vi "Instructor Read Client.vi"() -> ()   [LabVIEW 2017]
uses:
  <vilib>/OPCUA/controls/NodeIds.ctl
  <vilib>/OPCUA/controls/NodeId.ctl
  <vilib>/OPCUA/NI OPC UA Client.lvlib
panel:
  in  "stop":bool
  out "error out":errorcluster
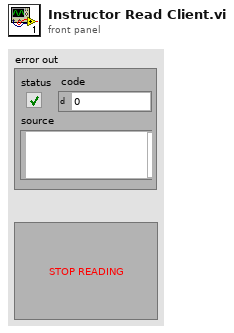
[diagram p1: front panel]
types:
  T1 = cluster{"message mode":enum16{"None", "Sign", "Sign and Encrypt"}, "security":enum16{"Basic256", "Basic128Rsa15"}}
  T2 = typedef "NodeIds.ctl" = T3[]
  T3 = typedef "NodeId.ctl" = string
  T4 = typedef "OPC UA Client Refnum.ctl" = refnum<k21>
  T5 = typedef "Subscription ID.ctl" = u32
  T6 = typedef "Subscription Data Change.ctl" = cluster{"node ID":T3, " value":variant, "timestamp":timestamp, "data type":T7, "status code":T8}
  T7 = typedef "Data Type.ctl" = u16
  T8 = typedef "OPC UA StatusCode.ctl" = u32
  T9 = cluster{"[0]":sgl, "[1]":sgl, "[2]":sgl, "[3]":sgl, "[4]":sgl, "[5]":sgl, "[6]":sgl, "[7]":sgl, "[8]":sgl, "[9]":sgl, "[10]":sgl, "[11]":sgl, "[12]":sgl, "[13]":sgl, "[14]":sgl, "[15]":sgl, "[16]":sgl, "[17]":sgl, "[18]":sgl, "[19]":sgl, "[20]":sgl, "[21]":sgl, "[22]":sgl, "[23]":sgl, "[24]":sgl, "[25]":sgl, "[26]":sgl, "[27]":sgl, "[28]":sgl, "[29]":sgl, "[30]":sgl, "[31]":sgl, "[32]":sgl, "[33]":sgl, "[34]":sgl, "[35]":sgl, "[36]":sgl, "[37]":sgl, "[38]":sgl, "[39]":sgl, "[40]":sgl, "[41]":sgl, "[42]":sgl, "[43]":sgl, "[44]":sgl, "[45]":sgl, "[46]":sgl, "[47]":sgl, "[48]":sgl, "[49]":sgl, "[50]":sgl, "[51]":sgl, "[52]":sgl, "[53]":sgl, "[54]":sgl, "[55]":sgl, "[56]":sgl, "[57]":sgl, "[58]":sgl, "[59]":sgl, "[60]":sgl, "[61]":sgl, "[62]":sgl}
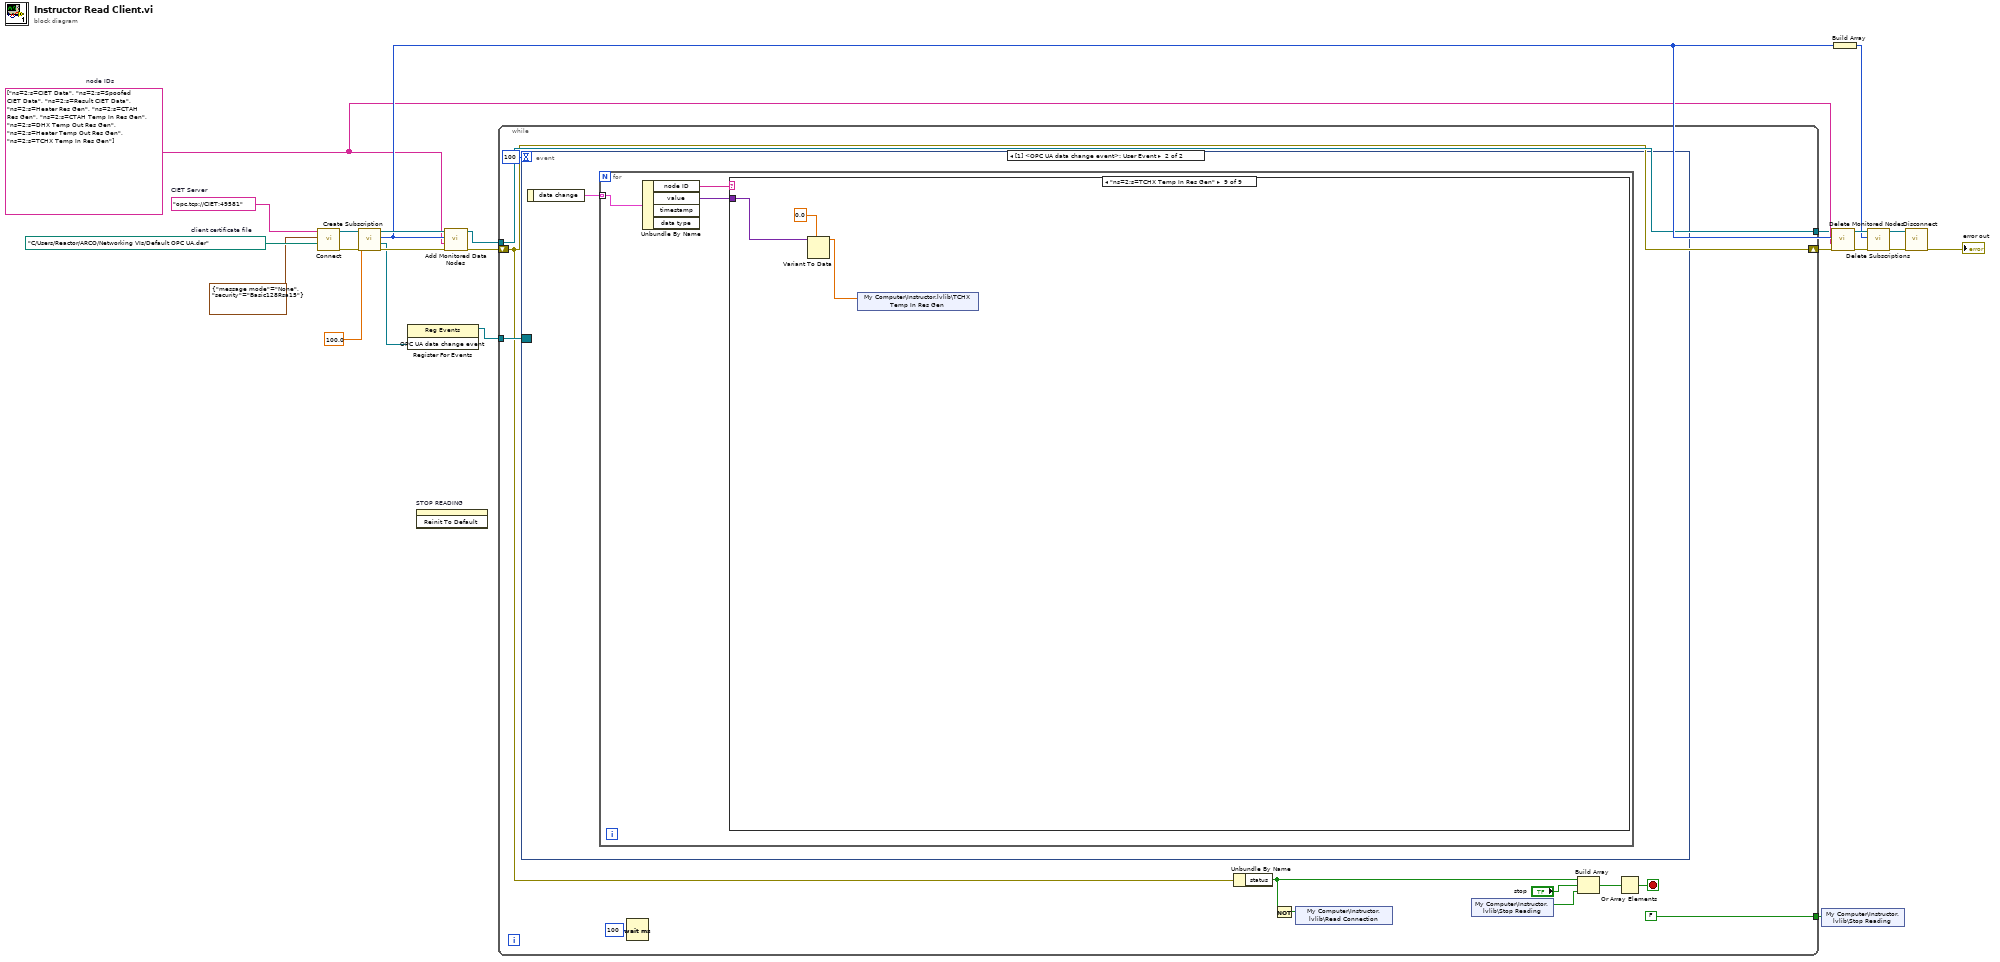
[diagram p0: block diagram]
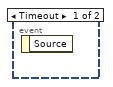
[diagram p2: hidden frame]
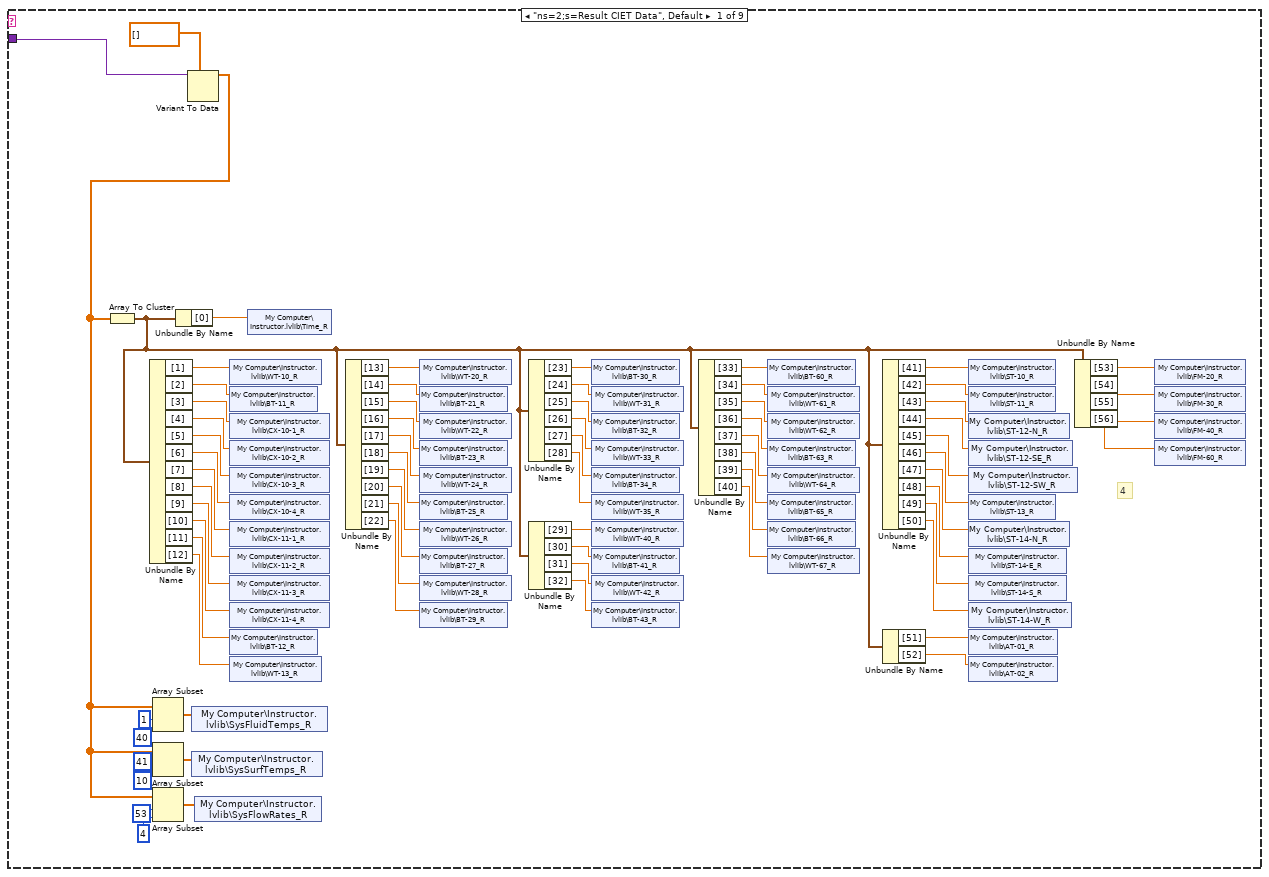
[diagram p3: hidden frame]
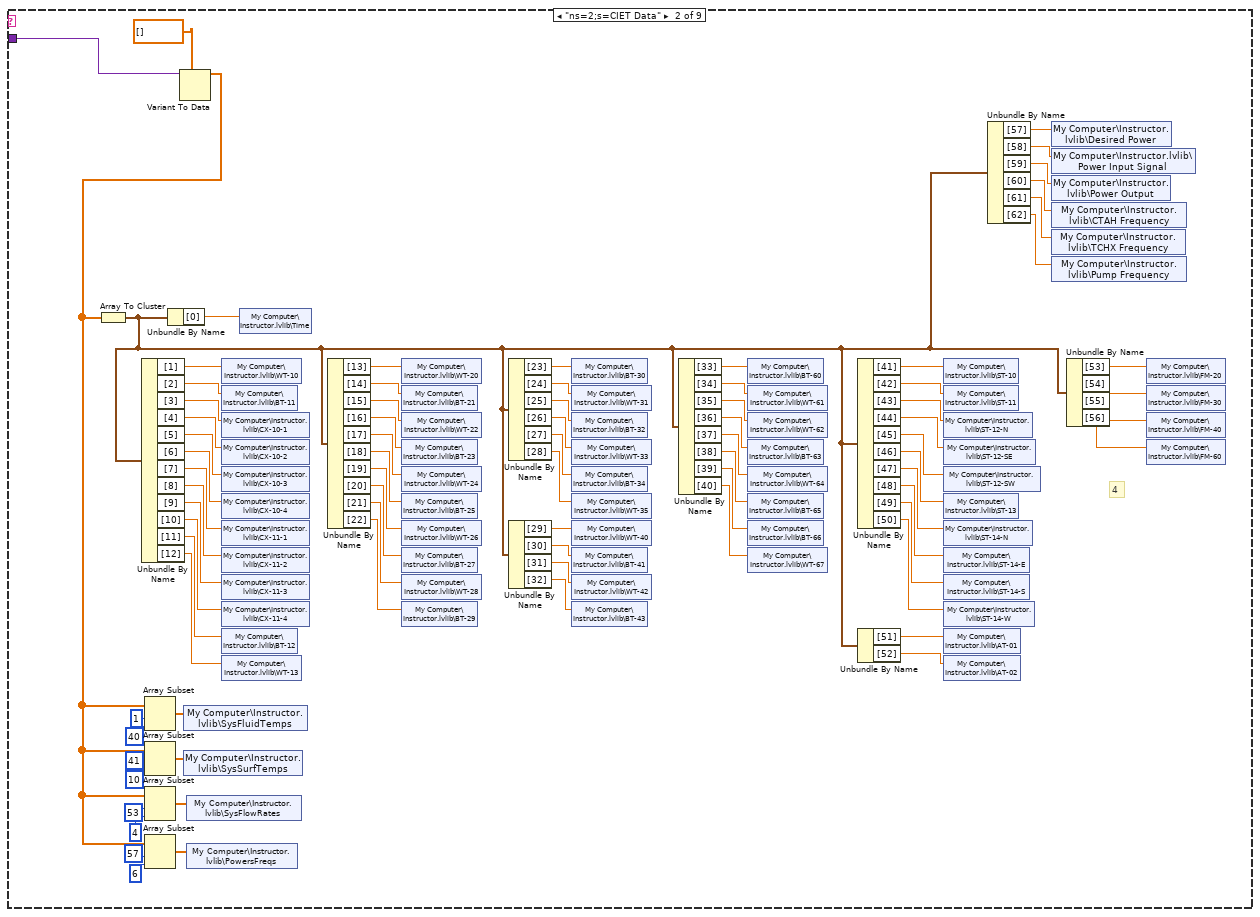
[diagram p4: hidden frame]
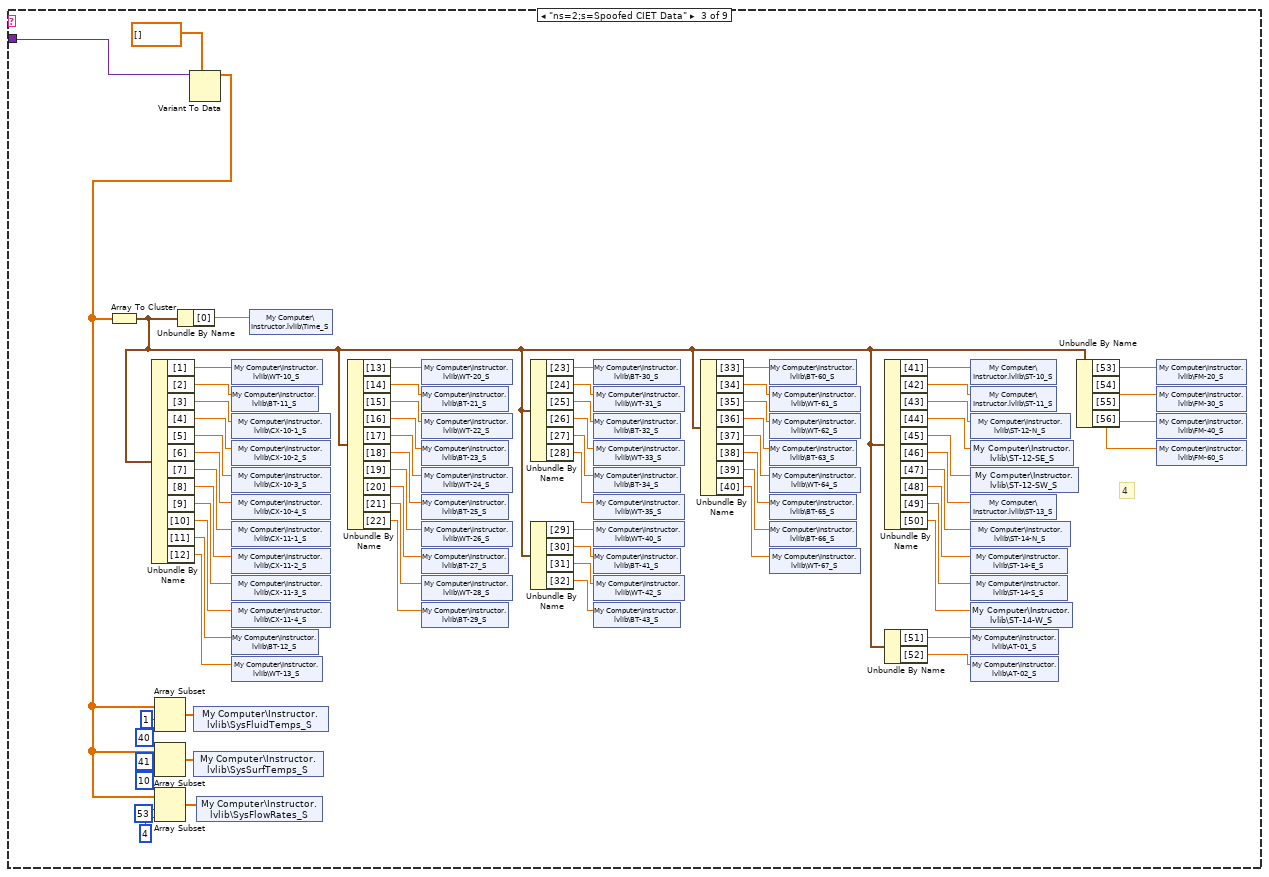
[diagram p5: hidden frame]
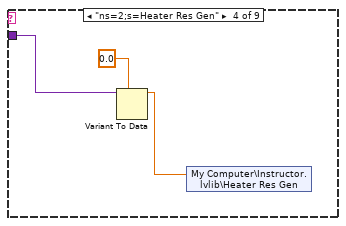
[diagram p6: hidden frame]
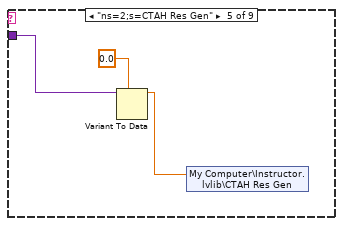
[diagram p7: hidden frame]
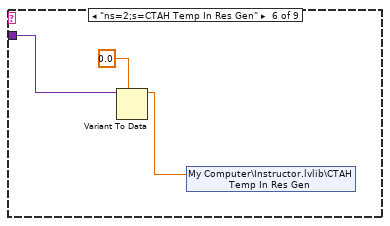
[diagram p8: hidden frame]
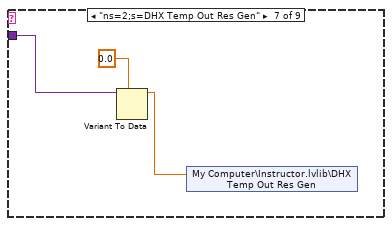
[diagram p9: hidden frame]
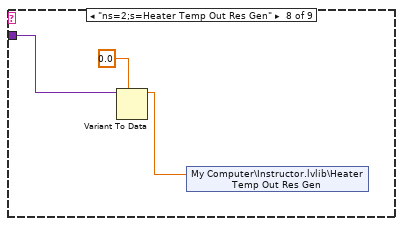
[diagram p10: hidden frame]
diagram:
  w7 = T2 ["ns=2;s=CIET Data", "ns=2;s=Spoofed CIET Data", "ns=2;s=Result CIET Data", "ns=2;s=Heater Res Gen", "ns=2;s=CTAH Res Gen", "ns=2;s=CTAH Temp In Res Gen", "ns=2;s=DHX Temp Out Res Gen", "ns=2;s=Heater Temp Out Res Gen", "ns=2;s=TCHX Temp In Res Gen"]  # node IDs
  w21 = path "C:/Users/Reactor/ARCO/Networking VIs/Default OPC UA.der"  # client certificate file
  w22 = "opc.tcp://CIET:49581"  # CIET Server
  n1 = call <vilib>:"Connect.vi"("client certificate file"=w21, "security policy"=T1 {"message mode"=enum."None", "security"=enum."Basic128Rsa15"}, "server endpoint URL"=w22) -> ("error out"=w3:errorcluster, "OPC UA client refnum out"=w19:T4)  [unwired: 6 in, 1 out]
  n2 = call <vilib>:"Create Subscription.vi"("error in (no error)"=w3, "publishing interval (1000 ms)"=100.0, "OPC UA client refnum in"=w19) -> ("error out"=w17:errorcluster, "OPC UA data change event"=w16:refnum<user-event>, "subscription ID out"=w11:T5, "OPC UA client refnum out"=w18:T4)  [unwired: 4 in, 1 out]
  n3 = register-events(w16) -> (reference out=w9:refnum<event-registration>)  [unwired: 2 in, 1 out]
  n4 = invoke on="STOP READING" class="Bool (strict)" method="Reinit To Default"() -> ()  [unwired: 3 in, 3 out]
  n5 = call <vilib>:"Add Monitored Data Nodes.vi"("error in (no error)"=w17, "node IDs"=w7, "subscription ID in"=w11, "OPC UA client refnum in"=w18) -> ("error out"=w2:errorcluster, "OPC UA client refnum out"=w8:T4)  [unwired: 4 in, 2 out]
  n6 = while {
    tunnel: w9 -> [w35]
    tunnel: w8 -> [w33]
    tunnel: [w33] -> w6
    tunnel: [FALSE] -> w4
    shift-right: [w24] -> w1
    shift-left: w2 -> [w24]
    stop <- w25 stop-if-true
    n7 = event shown="[1] <OPC UA data change event>: User Event" {
      selector: w35 -> [_ _]
      dyn-events: _ -> [_ _]
      timeout: 100 -> [_ _]
      event Timeout {
        n8 = event-data() -> ()  [unwired: 1 in, 1 out]
      }
      event User Event {
        n9 = event-data() -> ("data change"=w36:T6[])  [unwired: 1 in]
        n10 = for {
          tunnel: w36 -> [w38] mode=indexing
          n11 = Unbundle By Name(w38) -> ("node ID"=w37:T3, "value"=w39:variant)  [unwired: 2 out]
          n12 = case shown="\"ns=2;s=TCHX Temp In Res Gen\"" w37 {
            tunnel: w39 -> [w43 w129 w191 w259 w262 w265 w268 w271 w274]
            frame "ns=2;s=Result CIET Data", Default {
              # "4"
              n13 = Variant To Data(type=sgl[] [], Variant=w43) -> (data=w41:sgl[])  [unwired: 1 in, 1 out]
              n14 = Array To Cluster(array=w41) -> (cluster=w40:T9)
              n15 = Unbundle By Name(w40) -> ("[1]"=w50:sgl, "[2]"=w52:sgl, "[3]"=w53:sgl, "[4]"=w54:sgl, "[5]"=w55:sgl, "[6]"=w56:sgl, "[7]"=w57:sgl, "[8]"=w58:sgl, "[9]"=w59:sgl, "[10]"=w60:sgl, "[11]"=w61:sgl, "[12]"=w62:sgl)
              n16 = Array Subset(array=w41, index=1, length=40) -> (w107:sgl[])
              n17 = Array Subset(array=w41, index=41, length=10) -> (w108:sgl[])
              n18 = Array Subset(array=w41, index=53, length=4) -> (w109:sgl[])
              n19 = Unbundle By Name(w40) -> ("[0]"=w51:sgl)
              n20 = shared-variable "My Computer\\Instructor.lvlib\\SysFluidTemps_R"(w107) -> ()  [unwired: 1 in, 1 out]
              n21 = shared-variable "My Computer\\Instructor.lvlib\\SysSurfTemps_R"(w108) -> ()  [unwired: 1 in, 1 out]
              n22 = shared-variable "My Computer\\Instructor.lvlib\\SysFlowRates_R"(w109) -> ()  [unwired: 1 in, 1 out]
              n23 = shared-variable "My Computer\\Instructor.lvlib\\WT-10_R"(w50) -> ()  [unwired: 1 in, 1 out]
              n24 = shared-variable "My Computer\\Instructor.lvlib\\BT-11_R"(w52) -> ()  [unwired: 1 in, 1 out]
              n25 = shared-variable "My Computer\\Instructor.lvlib\\CX-10-1_R"(w53) -> ()  [unwired: 1 in, 1 out]
              n26 = shared-variable "My Computer\\Instructor.lvlib\\CX-10-2_R"(w54) -> ()  [unwired: 1 in, 1 out]
              n27 = shared-variable "My Computer\\Instructor.lvlib\\CX-10-3_R"(w55) -> ()  [unwired: 1 in, 1 out]
              n28 = shared-variable "My Computer\\Instructor.lvlib\\CX-10-4_R"(w56) -> ()  [unwired: 1 in, 1 out]
              n29 = shared-variable "My Computer\\Instructor.lvlib\\CX-11-1_R"(w57) -> ()  [unwired: 1 in, 1 out]
              n30 = shared-variable "My Computer\\Instructor.lvlib\\CX-11-2_R"(w58) -> ()  [unwired: 1 in, 1 out]
              n31 = shared-variable "My Computer\\Instructor.lvlib\\CX-11-3_R"(w59) -> ()  [unwired: 1 in, 1 out]
              n32 = shared-variable "My Computer\\Instructor.lvlib\\CX-11-4_R"(w60) -> ()  [unwired: 1 in, 1 out]
              n33 = shared-variable "My Computer\\Instructor.lvlib\\BT-12_R"(w61) -> ()  [unwired: 1 in, 1 out]
              n34 = shared-variable "My Computer\\Instructor.lvlib\\WT-13_R"(w62) -> ()  [unwired: 1 in, 1 out]
              n35 = shared-variable "My Computer\\Instructor.lvlib\\Time_R"(w51) -> ()  [unwired: 1 in, 1 out]
              n36 = Unbundle By Name(w40) -> ("[13]"=w63:sgl, "[14]"=w64:sgl, "[15]"=w65:sgl, "[16]"=w66:sgl, "[17]"=w67:sgl, "[18]"=w68:sgl, "[19]"=w69:sgl, "[20]"=w70:sgl, "[21]"=w71:sgl, "[22]"=w72:sgl)
              n37 = shared-variable "My Computer\\Instructor.lvlib\\WT-20_R"(w63) -> ()  [unwired: 1 in, 1 out]
              n38 = shared-variable "My Computer\\Instructor.lvlib\\BT-21_R"(w64) -> ()  [unwired: 1 in, 1 out]
              n39 = shared-variable "My Computer\\Instructor.lvlib\\WT-22_R"(w65) -> ()  [unwired: 1 in, 1 out]
              n40 = shared-variable "My Computer\\Instructor.lvlib\\BT-23_R"(w66) -> ()  [unwired: 1 in, 1 out]
              n41 = shared-variable "My Computer\\Instructor.lvlib\\WT-24_R"(w67) -> ()  [unwired: 1 in, 1 out]
              n42 = shared-variable "My Computer\\Instructor.lvlib\\BT-25_R"(w68) -> ()  [unwired: 1 in, 1 out]
              n43 = shared-variable "My Computer\\Instructor.lvlib\\WT-26_R"(w69) -> ()  [unwired: 1 in, 1 out]
              n44 = shared-variable "My Computer\\Instructor.lvlib\\BT-27_R"(w70) -> ()  [unwired: 1 in, 1 out]
              n45 = shared-variable "My Computer\\Instructor.lvlib\\WT-28_R"(w71) -> ()  [unwired: 1 in, 1 out]
              n46 = shared-variable "My Computer\\Instructor.lvlib\\BT-29_R"(w72) -> ()  [unwired: 1 in, 1 out]
              n47 = Unbundle By Name(w40) -> ("[23]"=w73:sgl, "[24]"=w74:sgl, "[25]"=w75:sgl, "[26]"=w76:sgl, "[27]"=w77:sgl, "[28]"=w78:sgl)
              n48 = Unbundle By Name(w40) -> ("[29]"=w79:sgl, "[30]"=w80:sgl, "[31]"=w81:sgl, "[32]"=w82:sgl)
              n49 = shared-variable "My Computer\\Instructor.lvlib\\BT-30_R"(w73) -> ()  [unwired: 1 in, 1 out]
              n50 = shared-variable "My Computer\\Instructor.lvlib\\WT-31_R"(w74) -> ()  [unwired: 1 in, 1 out]
              n51 = shared-variable "My Computer\\Instructor.lvlib\\BT-32_R"(w75) -> ()  [unwired: 1 in, 1 out]
              n52 = shared-variable "My Computer\\Instructor.lvlib\\WT-33_R"(w76) -> ()  [unwired: 1 in, 1 out]
              n53 = shared-variable "My Computer\\Instructor.lvlib\\BT-34_R"(w77) -> ()  [unwired: 1 in, 1 out]
              n54 = shared-variable "My Computer\\Instructor.lvlib\\WT-35_R"(w78) -> ()  [unwired: 1 in, 1 out]
              n55 = shared-variable "My Computer\\Instructor.lvlib\\WT-40_R"(w79) -> ()  [unwired: 1 in, 1 out]
              n56 = shared-variable "My Computer\\Instructor.lvlib\\BT-41_R"(w80) -> ()  [unwired: 1 in, 1 out]
              n57 = shared-variable "My Computer\\Instructor.lvlib\\WT-42_R"(w81) -> ()  [unwired: 1 in, 1 out]
              n58 = shared-variable "My Computer\\Instructor.lvlib\\BT-43_R"(w82) -> ()  [unwired: 1 in, 1 out]
              n59 = Unbundle By Name(w40) -> ("[33]"=w83:sgl, "[34]"=w84:sgl, "[35]"=w85:sgl, "[36]"=w86:sgl, "[37]"=w87:sgl, "[38]"=w88:sgl, "[39]"=w89:sgl, "[40]"=w90:sgl)
              n60 = shared-variable "My Computer\\Instructor.lvlib\\BT-60_R"(w83) -> ()  [unwired: 1 in, 1 out]
              n61 = shared-variable "My Computer\\Instructor.lvlib\\WT-61_R"(w84) -> ()  [unwired: 1 in, 1 out]
              n62 = shared-variable "My Computer\\Instructor.lvlib\\WT-62_R"(w85) -> ()  [unwired: 1 in, 1 out]
              n63 = shared-variable "My Computer\\Instructor.lvlib\\BT-63_R"(w86) -> ()  [unwired: 1 in, 1 out]
              n64 = shared-variable "My Computer\\Instructor.lvlib\\WT-64_R"(w87) -> ()  [unwired: 1 in, 1 out]
              n65 = shared-variable "My Computer\\Instructor.lvlib\\BT-65_R"(w88) -> ()  [unwired: 1 in, 1 out]
              n66 = shared-variable "My Computer\\Instructor.lvlib\\BT-66_R"(w89) -> ()  [unwired: 1 in, 1 out]
              n67 = shared-variable "My Computer\\Instructor.lvlib\\WT-67_R"(w90) -> ()  [unwired: 1 in, 1 out]
              n68 = Unbundle By Name(w40) -> ("[41]"=w91:sgl, "[42]"=w92:sgl, "[43]"=w93:sgl, "[44]"=w94:sgl, "[45]"=w95:sgl, "[46]"=w96:sgl, "[47]"=w97:sgl, "[48]"=w98:sgl, "[49]"=w99:sgl, "[50]"=w100:sgl)
              n69 = Unbundle By Name(w40) -> ("[51]"=w101:sgl, "[52]"=w102:sgl)
              n70 = shared-variable "My Computer\\Instructor.lvlib\\ST-10_R"(w91) -> ()  [unwired: 1 in, 1 out]
              n71 = shared-variable "My Computer\\Instructor.lvlib\\ST-11_R"(w92) -> ()  [unwired: 1 in, 1 out]
              n72 = shared-variable "My Computer\\Instructor.lvlib\\ST-12-N_R"(w93) -> ()  [unwired: 1 in, 1 out]
              n73 = shared-variable "My Computer\\Instructor.lvlib\\ST-12-SE_R"(w94) -> ()  [unwired: 1 in, 1 out]
              n74 = shared-variable "My Computer\\Instructor.lvlib\\ST-12-SW_R"(w95) -> ()  [unwired: 1 in, 1 out]
              n75 = shared-variable "My Computer\\Instructor.lvlib\\ST-13_R"(w96) -> ()  [unwired: 1 in, 1 out]
              n76 = shared-variable "My Computer\\Instructor.lvlib\\ST-14-N_R"(w97) -> ()  [unwired: 1 in, 1 out]
              n77 = shared-variable "My Computer\\Instructor.lvlib\\ST-14-E_R"(w98) -> ()  [unwired: 1 in, 1 out]
              n78 = shared-variable "My Computer\\Instructor.lvlib\\ST-14-S_R"(w99) -> ()  [unwired: 1 in, 1 out]
              n79 = shared-variable "My Computer\\Instructor.lvlib\\ST-14-W_R"(w100) -> ()  [unwired: 1 in, 1 out]
              n80 = shared-variable "My Computer\\Instructor.lvlib\\AT-01_R"(w101) -> ()  [unwired: 1 in, 1 out]
              n81 = shared-variable "My Computer\\Instructor.lvlib\\AT-02_R"(w102) -> ()  [unwired: 1 in, 1 out]
              n82 = Unbundle By Name(w40) -> ("[53]"=w103:sgl, "[54]"=w104:sgl, "[55]"=w105:sgl, "[56]"=w106:sgl)
              n83 = shared-variable "My Computer\\Instructor.lvlib\\FM-20_R"(w103) -> ()  [unwired: 1 in, 1 out]
              n84 = shared-variable "My Computer\\Instructor.lvlib\\FM-30_R"(w104) -> ()  [unwired: 1 in, 1 out]
              n85 = shared-variable "My Computer\\Instructor.lvlib\\FM-40_R"(w105) -> ()  [unwired: 1 in, 1 out]
              n86 = shared-variable "My Computer\\Instructor.lvlib\\FM-60_R"(w106) -> ()  [unwired: 1 in, 1 out]
            }
            frame "ns=2;s=CIET Data" {
              # "4"
              n87 = Variant To Data(type=sgl[] [], Variant=w129) -> (data=w111:sgl[])  [unwired: 1 in, 1 out]
              n88 = Array To Cluster(array=w111) -> (cluster=w110:T9)
              n89 = Unbundle By Name(w110) -> ("[1]"=w128:sgl, "[2]"=w131:sgl, "[3]"=w132:sgl, "[4]"=w133:sgl, "[5]"=w134:sgl, "[6]"=w135:sgl, "[7]"=w136:sgl, "[8]"=w137:sgl, "[9]"=w138:sgl, "[10]"=w139:sgl, "[11]"=w140:sgl, "[12]"=w141:sgl)
              n90 = Array Subset(array=w111, index=1, length=40) -> (w186:sgl[])
              n91 = Array Subset(array=w111, index=41, length=10) -> (w187:sgl[])
              n92 = Array Subset(array=w111, index=53, length=4) -> (w188:sgl[])
              n93 = Array Subset(array=w111, index=57, length=6) -> (w118:sgl[])
              n94 = Unbundle By Name(w110) -> ("[0]"=w130:sgl)
              n95 = shared-variable "My Computer\\Instructor.lvlib\\SysFluidTemps"(w186) -> ()  [unwired: 1 in, 1 out]
              n96 = shared-variable "My Computer\\Instructor.lvlib\\SysSurfTemps"(w187) -> ()  [unwired: 1 in, 1 out]
              n97 = shared-variable "My Computer\\Instructor.lvlib\\SysFlowRates"(w188) -> ()  [unwired: 1 in, 1 out]
              n98 = shared-variable "My Computer\\Instructor.lvlib\\PowersFreqs"(w118) -> ()  [unwired: 1 in, 1 out]
              n99 = shared-variable "My Computer\\Instructor.lvlib\\WT-10"(w128) -> ()  [unwired: 1 in, 1 out]
              n100 = shared-variable "My Computer\\Instructor.lvlib\\BT-11"(w131) -> ()  [unwired: 1 in, 1 out]
              n101 = shared-variable "My Computer\\Instructor.lvlib\\CX-10-1"(w132) -> ()  [unwired: 1 in, 1 out]
              n102 = shared-variable "My Computer\\Instructor.lvlib\\CX-10-2"(w133) -> ()  [unwired: 1 in, 1 out]
              n103 = shared-variable "My Computer\\Instructor.lvlib\\CX-10-3"(w134) -> ()  [unwired: 1 in, 1 out]
              n104 = shared-variable "My Computer\\Instructor.lvlib\\CX-10-4"(w135) -> ()  [unwired: 1 in, 1 out]
              n105 = shared-variable "My Computer\\Instructor.lvlib\\CX-11-1"(w136) -> ()  [unwired: 1 in, 1 out]
              n106 = shared-variable "My Computer\\Instructor.lvlib\\CX-11-2"(w137) -> ()  [unwired: 1 in, 1 out]
              n107 = shared-variable "My Computer\\Instructor.lvlib\\CX-11-3"(w138) -> ()  [unwired: 1 in, 1 out]
              n108 = shared-variable "My Computer\\Instructor.lvlib\\CX-11-4"(w139) -> ()  [unwired: 1 in, 1 out]
              n109 = shared-variable "My Computer\\Instructor.lvlib\\BT-12"(w140) -> ()  [unwired: 1 in, 1 out]
              n110 = shared-variable "My Computer\\Instructor.lvlib\\WT-13"(w141) -> ()  [unwired: 1 in, 1 out]
              n111 = shared-variable "My Computer\\Instructor.lvlib\\Time"(w130) -> ()  [unwired: 1 in, 1 out]
              n112 = Unbundle By Name(w110) -> ("[13]"=w142:sgl, "[14]"=w143:sgl, "[15]"=w144:sgl, "[16]"=w145:sgl, "[17]"=w146:sgl, "[18]"=w147:sgl, "[19]"=w148:sgl, "[20]"=w149:sgl, "[21]"=w150:sgl, "[22]"=w151:sgl)
              n113 = shared-variable "My Computer\\Instructor.lvlib\\WT-20"(w142) -> ()  [unwired: 1 in, 1 out]
              n114 = shared-variable "My Computer\\Instructor.lvlib\\BT-21"(w143) -> ()  [unwired: 1 in, 1 out]
              n115 = shared-variable "My Computer\\Instructor.lvlib\\WT-22"(w144) -> ()  [unwired: 1 in, 1 out]
              n116 = shared-variable "My Computer\\Instructor.lvlib\\BT-23"(w145) -> ()  [unwired: 1 in, 1 out]
              n117 = shared-variable "My Computer\\Instructor.lvlib\\WT-24"(w146) -> ()  [unwired: 1 in, 1 out]
              n118 = shared-variable "My Computer\\Instructor.lvlib\\BT-25"(w147) -> ()  [unwired: 1 in, 1 out]
              n119 = shared-variable "My Computer\\Instructor.lvlib\\WT-26"(w148) -> ()  [unwired: 1 in, 1 out]
              n120 = shared-variable "My Computer\\Instructor.lvlib\\BT-27"(w149) -> ()  [unwired: 1 in, 1 out]
              n121 = shared-variable "My Computer\\Instructor.lvlib\\WT-28"(w150) -> ()  [unwired: 1 in, 1 out]
              n122 = shared-variable "My Computer\\Instructor.lvlib\\BT-29"(w151) -> ()  [unwired: 1 in, 1 out]
              n123 = Unbundle By Name(w110) -> ("[23]"=w152:sgl, "[24]"=w153:sgl, "[25]"=w154:sgl, "[26]"=w155:sgl, "[27]"=w156:sgl, "[28]"=w157:sgl)
              n124 = Unbundle By Name(w110) -> ("[29]"=w158:sgl, "[30]"=w159:sgl, "[31]"=w160:sgl, "[32]"=w161:sgl)
              n125 = shared-variable "My Computer\\Instructor.lvlib\\BT-30"(w152) -> ()  [unwired: 1 in, 1 out]
              n126 = shared-variable "My Computer\\Instructor.lvlib\\WT-31"(w153) -> ()  [unwired: 1 in, 1 out]
              n127 = shared-variable "My Computer\\Instructor.lvlib\\BT-32"(w154) -> ()  [unwired: 1 in, 1 out]
              n128 = shared-variable "My Computer\\Instructor.lvlib\\WT-33"(w155) -> ()  [unwired: 1 in, 1 out]
              n129 = shared-variable "My Computer\\Instructor.lvlib\\BT-34"(w156) -> ()  [unwired: 1 in, 1 out]
              n130 = shared-variable "My Computer\\Instructor.lvlib\\WT-35"(w157) -> ()  [unwired: 1 in, 1 out]
              n131 = shared-variable "My Computer\\Instructor.lvlib\\WT-40"(w158) -> ()  [unwired: 1 in, 1 out]
              n132 = shared-variable "My Computer\\Instructor.lvlib\\BT-41"(w159) -> ()  [unwired: 1 in, 1 out]
              n133 = shared-variable "My Computer\\Instructor.lvlib\\WT-42"(w160) -> ()  [unwired: 1 in, 1 out]
              n134 = shared-variable "My Computer\\Instructor.lvlib\\BT-43"(w161) -> ()  [unwired: 1 in, 1 out]
              n135 = Unbundle By Name(w110) -> ("[33]"=w162:sgl, "[34]"=w163:sgl, "[35]"=w164:sgl, "[36]"=w165:sgl, "[37]"=w166:sgl, "[38]"=w167:sgl, "[39]"=w168:sgl, "[40]"=w169:sgl)
              n136 = shared-variable "My Computer\\Instructor.lvlib\\BT-60"(w162) -> ()  [unwired: 1 in, 1 out]
              n137 = shared-variable "My Computer\\Instructor.lvlib\\WT-61"(w163) -> ()  [unwired: 1 in, 1 out]
              n138 = shared-variable "My Computer\\Instructor.lvlib\\WT-62"(w164) -> ()  [unwired: 1 in, 1 out]
              n139 = shared-variable "My Computer\\Instructor.lvlib\\BT-63"(w165) -> ()  [unwired: 1 in, 1 out]
              n140 = shared-variable "My Computer\\Instructor.lvlib\\WT-64"(w166) -> ()  [unwired: 1 in, 1 out]
              n141 = shared-variable "My Computer\\Instructor.lvlib\\BT-65"(w167) -> ()  [unwired: 1 in, 1 out]
              n142 = shared-variable "My Computer\\Instructor.lvlib\\BT-66"(w168) -> ()  [unwired: 1 in, 1 out]
              n143 = shared-variable "My Computer\\Instructor.lvlib\\WT-67"(w169) -> ()  [unwired: 1 in, 1 out]
              n144 = Unbundle By Name(w110) -> ("[41]"=w170:sgl, "[42]"=w171:sgl, "[43]"=w172:sgl, "[44]"=w173:sgl, "[45]"=w174:sgl, "[46]"=w175:sgl, "[47]"=w176:sgl, "[48]"=w177:sgl, "[49]"=w178:sgl, "[50]"=w179:sgl)
              n145 = Unbundle By Name(w110) -> ("[51]"=w180:sgl, "[52]"=w181:sgl)
              n146 = shared-variable "My Computer\\Instructor.lvlib\\ST-10"(w170) -> ()  [unwired: 1 in, 1 out]
              n147 = shared-variable "My Computer\\Instructor.lvlib\\ST-11"(w171) -> ()  [unwired: 1 in, 1 out]
              n148 = shared-variable "My Computer\\Instructor.lvlib\\ST-12-N"(w172) -> ()  [unwired: 1 in, 1 out]
              n149 = shared-variable "My Computer\\Instructor.lvlib\\ST-12-SE"(w173) -> ()  [unwired: 1 in, 1 out]
              n150 = shared-variable "My Computer\\Instructor.lvlib\\ST-12-SW"(w174) -> ()  [unwired: 1 in, 1 out]
              n151 = shared-variable "My Computer\\Instructor.lvlib\\ST-13"(w175) -> ()  [unwired: 1 in, 1 out]
              n152 = shared-variable "My Computer\\Instructor.lvlib\\ST-14-N"(w176) -> ()  [unwired: 1 in, 1 out]
              n153 = shared-variable "My Computer\\Instructor.lvlib\\ST-14-E"(w177) -> ()  [unwired: 1 in, 1 out]
              n154 = shared-variable "My Computer\\Instructor.lvlib\\ST-14-S"(w178) -> ()  [unwired: 1 in, 1 out]
              n155 = shared-variable "My Computer\\Instructor.lvlib\\ST-14-W"(w179) -> ()  [unwired: 1 in, 1 out]
              n156 = shared-variable "My Computer\\Instructor.lvlib\\AT-01"(w180) -> ()  [unwired: 1 in, 1 out]
              n157 = shared-variable "My Computer\\Instructor.lvlib\\AT-02"(w181) -> ()  [unwired: 1 in, 1 out]
              n158 = Unbundle By Name(w110) -> ("[57]"=w117:sgl, "[58]"=w116:sgl, "[59]"=w115:sgl, "[60]"=w114:sgl, "[61]"=w113:sgl, "[62]"=w112:sgl)
              n159 = shared-variable "My Computer\\Instructor.lvlib\\Desired Power"(w117) -> ()  [unwired: 1 in, 1 out]
              n160 = shared-variable "My Computer\\Instructor.lvlib\\Power Input Signal"(w116) -> ()  [unwired: 1 in, 1 out]
              n161 = shared-variable "My Computer\\Instructor.lvlib\\Power Output"(w115) -> ()  [unwired: 1 in, 1 out]
              n162 = shared-variable "My Computer\\Instructor.lvlib\\CTAH Frequency"(w114) -> ()  [unwired: 1 in, 1 out]
              n163 = shared-variable "My Computer\\Instructor.lvlib\\TCHX Frequency"(w113) -> ()  [unwired: 1 in, 1 out]
              n164 = shared-variable "My Computer\\Instructor.lvlib\\Pump Frequency"(w112) -> ()  [unwired: 1 in, 1 out]
              n165 = Unbundle By Name(w110) -> ("[53]"=w182:sgl, "[54]"=w183:sgl, "[55]"=w184:sgl, "[56]"=w185:sgl)
              n166 = shared-variable "My Computer\\Instructor.lvlib\\FM-20"(w182) -> ()  [unwired: 1 in, 1 out]
              n167 = shared-variable "My Computer\\Instructor.lvlib\\FM-30"(w183) -> ()  [unwired: 1 in, 1 out]
              n168 = shared-variable "My Computer\\Instructor.lvlib\\FM-40"(w184) -> ()  [unwired: 1 in, 1 out]
              n169 = shared-variable "My Computer\\Instructor.lvlib\\FM-60"(w185) -> ()  [unwired: 1 in, 1 out]
            }
            frame "ns=2;s=Spoofed CIET Data" {
              # "4"
              n170 = Variant To Data(type=sgl[] [], Variant=w191) -> (data=w190:sgl[])  [unwired: 1 in, 1 out]
              n171 = Array To Cluster(array=w190) -> (cluster=w189:T9)
              n172 = Unbundle By Name(w189) -> ("[1]"=w199:sgl, "[2]"=w201:sgl, "[3]"=w202:sgl, "[4]"=w203:sgl, "[5]"=w204:sgl, "[6]"=w205:sgl, "[7]"=w206:sgl, "[8]"=w207:sgl, "[9]"=w208:sgl, "[10]"=w209:sgl, "[11]"=w210:sgl, "[12]"=w211:sgl)
              n173 = Array Subset(array=w190, index=1, length=40) -> (w256:sgl[])
              n174 = Array Subset(array=w190, index=41, length=10) -> (w257:sgl[])
              n175 = Array Subset(array=w190, index=53, length=4) -> (w258:sgl[])
              n176 = Unbundle By Name(w189) -> ("[0]"=w200:sgl)
              n177 = shared-variable "My Computer\\Instructor.lvlib\\SysFluidTemps_S"(w256) -> ()  [unwired: 1 in, 1 out]
              n178 = shared-variable "My Computer\\Instructor.lvlib\\SysSurfTemps_S"(w257) -> ()  [unwired: 1 in, 1 out]
              n179 = shared-variable "My Computer\\Instructor.lvlib\\SysFlowRates_S"(w258) -> ()  [unwired: 1 in, 1 out]
              n180 = shared-variable "My Computer\\Instructor.lvlib\\WT-10_S"(w199) -> ()  [unwired: 1 in, 1 out]
              n181 = shared-variable "My Computer\\Instructor.lvlib\\BT-11_S"(w201) -> ()  [unwired: 1 in, 1 out]
              n182 = shared-variable "My Computer\\Instructor.lvlib\\CX-10-1_S"(w202) -> ()  [unwired: 1 in, 1 out]
              n183 = shared-variable "My Computer\\Instructor.lvlib\\CX-10-2_S"(w203) -> ()  [unwired: 1 in, 1 out]
              n184 = shared-variable "My Computer\\Instructor.lvlib\\CX-10-3_S"(w204) -> ()  [unwired: 1 in, 1 out]
              n185 = shared-variable "My Computer\\Instructor.lvlib\\CX-10-4_S"(w205) -> ()  [unwired: 1 in, 1 out]
              n186 = shared-variable "My Computer\\Instructor.lvlib\\CX-11-1_S"(w206) -> ()  [unwired: 1 in, 1 out]
              n187 = shared-variable "My Computer\\Instructor.lvlib\\CX-11-2_S"(w207) -> ()  [unwired: 1 in, 1 out]
              n188 = shared-variable "My Computer\\Instructor.lvlib\\CX-11-3_S"(w208) -> ()  [unwired: 1 in, 1 out]
              n189 = shared-variable "My Computer\\Instructor.lvlib\\CX-11-4_S"(w209) -> ()  [unwired: 1 in, 1 out]
              n190 = shared-variable "My Computer\\Instructor.lvlib\\BT-12_S"(w210) -> ()  [unwired: 1 in, 1 out]
              n191 = shared-variable "My Computer\\Instructor.lvlib\\WT-13_S"(w211) -> ()  [unwired: 1 in, 1 out]
              n192 = shared-variable "My Computer\\Instructor.lvlib\\Time_S"(w200) -> ()  [unwired: 1 in, 1 out]
              n193 = Unbundle By Name(w189) -> ("[13]"=w212:sgl, "[14]"=w213:sgl, "[15]"=w214:sgl, "[16]"=w215:sgl, "[17]"=w216:sgl, "[18]"=w217:sgl, "[19]"=w218:sgl, "[20]"=w219:sgl, "[21]"=w220:sgl, "[22]"=w221:sgl)
              n194 = shared-variable "My Computer\\Instructor.lvlib\\WT-20_S"(w212) -> ()  [unwired: 1 in, 1 out]
              n195 = shared-variable "My Computer\\Instructor.lvlib\\BT-21_S"(w213) -> ()  [unwired: 1 in, 1 out]
              n196 = shared-variable "My Computer\\Instructor.lvlib\\WT-22_S"(w214) -> ()  [unwired: 1 in, 1 out]
              n197 = shared-variable "My Computer\\Instructor.lvlib\\BT-23_S"(w215) -> ()  [unwired: 1 in, 1 out]
              n198 = shared-variable "My Computer\\Instructor.lvlib\\WT-24_S"(w216) -> ()  [unwired: 1 in, 1 out]
              n199 = shared-variable "My Computer\\Instructor.lvlib\\BT-25_S"(w217) -> ()  [unwired: 1 in, 1 out]
              n200 = shared-variable "My Computer\\Instructor.lvlib\\WT-26_S"(w218) -> ()  [unwired: 1 in, 1 out]
              n201 = shared-variable "My Computer\\Instructor.lvlib\\BT-27_S"(w219) -> ()  [unwired: 1 in, 1 out]
              n202 = shared-variable "My Computer\\Instructor.lvlib\\WT-28_S"(w220) -> ()  [unwired: 1 in, 1 out]
              n203 = shared-variable "My Computer\\Instructor.lvlib\\BT-29_S"(w221) -> ()  [unwired: 1 in, 1 out]
              n204 = Unbundle By Name(w189) -> ("[23]"=w222:sgl, "[24]"=w223:sgl, "[25]"=w224:sgl, "[26]"=w225:sgl, "[27]"=w226:sgl, "[28]"=w227:sgl)
              n205 = Unbundle By Name(w189) -> ("[29]"=w228:sgl, "[30]"=w229:sgl, "[31]"=w230:sgl, "[32]"=w231:sgl)
              n206 = shared-variable "My Computer\\Instructor.lvlib\\BT-30_S"(w222) -> ()  [unwired: 1 in, 1 out]
              n207 = shared-variable "My Computer\\Instructor.lvlib\\WT-31_S"(w223) -> ()  [unwired: 1 in, 1 out]
              n208 = shared-variable "My Computer\\Instructor.lvlib\\BT-32_S"(w224) -> ()  [unwired: 1 in, 1 out]
              n209 = shared-variable "My Computer\\Instructor.lvlib\\WT-33_S"(w225) -> ()  [unwired: 1 in, 1 out]
              n210 = shared-variable "My Computer\\Instructor.lvlib\\BT-34_S"(w226) -> ()  [unwired: 1 in, 1 out]
              n211 = shared-variable "My Computer\\Instructor.lvlib\\WT-35_S"(w227) -> ()  [unwired: 1 in, 1 out]
              n212 = shared-variable "My Computer\\Instructor.lvlib\\WT-40_S"(w228) -> ()  [unwired: 1 in, 1 out]
              n213 = shared-variable "My Computer\\Instructor.lvlib\\BT-41_S"(w229) -> ()  [unwired: 1 in, 1 out]
              n214 = shared-variable "My Computer\\Instructor.lvlib\\WT-42_S"(w230) -> ()  [unwired: 1 in, 1 out]
              n215 = shared-variable "My Computer\\Instructor.lvlib\\BT-43_S"(w231) -> ()  [unwired: 1 in, 1 out]
              n216 = Unbundle By Name(w189) -> ("[33]"=w232:sgl, "[34]"=w233:sgl, "[35]"=w234:sgl, "[36]"=w235:sgl, "[37]"=w236:sgl, "[38]"=w237:sgl, "[39]"=w238:sgl, "[40]"=w239:sgl)
              n217 = shared-variable "My Computer\\Instructor.lvlib\\BT-60_S"(w232) -> ()  [unwired: 1 in, 1 out]
              n218 = shared-variable "My Computer\\Instructor.lvlib\\WT-61_S"(w233) -> ()  [unwired: 1 in, 1 out]
              n219 = shared-variable "My Computer\\Instructor.lvlib\\WT-62_S"(w234) -> ()  [unwired: 1 in, 1 out]
              n220 = shared-variable "My Computer\\Instructor.lvlib\\BT-63_S"(w235) -> ()  [unwired: 1 in, 1 out]
              n221 = shared-variable "My Computer\\Instructor.lvlib\\WT-64_S"(w236) -> ()  [unwired: 1 in, 1 out]
              n222 = shared-variable "My Computer\\Instructor.lvlib\\BT-65_S"(w237) -> ()  [unwired: 1 in, 1 out]
              n223 = shared-variable "My Computer\\Instructor.lvlib\\BT-66_S"(w238) -> ()  [unwired: 1 in, 1 out]
              n224 = shared-variable "My Computer\\Instructor.lvlib\\WT-67_S"(w239) -> ()  [unwired: 1 in, 1 out]
              n225 = Unbundle By Name(w189) -> ("[41]"=w240:sgl, "[42]"=w241:sgl, "[43]"=w242:sgl, "[44]"=w243:sgl, "[45]"=w244:sgl, "[46]"=w245:sgl, "[47]"=w246:sgl, "[48]"=w247:sgl, "[49]"=w248:sgl, "[50]"=w249:sgl)
              n226 = Unbundle By Name(w189) -> ("[51]"=w250:sgl, "[52]"=w251:sgl)
              n227 = shared-variable "My Computer\\Instructor.lvlib\\ST-10_S"(w240) -> ()  [unwired: 1 in, 1 out]
              n228 = shared-variable "My Computer\\Instructor.lvlib\\ST-11_S"(w241) -> ()  [unwired: 1 in, 1 out]
              n229 = shared-variable "My Computer\\Instructor.lvlib\\ST-12-N_S"(w242) -> ()  [unwired: 1 in, 1 out]
              n230 = shared-variable "My Computer\\Instructor.lvlib\\ST-12-SE_S"(w243) -> ()  [unwired: 1 in, 1 out]
              n231 = shared-variable "My Computer\\Instructor.lvlib\\ST-12-SW_S"(w244) -> ()  [unwired: 1 in, 1 out]
              n232 = shared-variable "My Computer\\Instructor.lvlib\\ST-13_S"(w245) -> ()  [unwired: 1 in, 1 out]
              n233 = shared-variable "My Computer\\Instructor.lvlib\\ST-14-N_S"(w246) -> ()  [unwired: 1 in, 1 out]
              n234 = shared-variable "My Computer\\Instructor.lvlib\\ST-14-E_S"(w247) -> ()  [unwired: 1 in, 1 out]
              n235 = shared-variable "My Computer\\Instructor.lvlib\\ST-14-S_S"(w248) -> ()  [unwired: 1 in, 1 out]
              n236 = shared-variable "My Computer\\Instructor.lvlib\\ST-14-W_S"(w249) -> ()  [unwired: 1 in, 1 out]
              n237 = shared-variable "My Computer\\Instructor.lvlib\\AT-01_S"(w250) -> ()  [unwired: 1 in, 1 out]
              n238 = shared-variable "My Computer\\Instructor.lvlib\\AT-02_S"(w251) -> ()  [unwired: 1 in, 1 out]
              n239 = Unbundle By Name(w189) -> ("[53]"=w252:sgl, "[54]"=w253:sgl, "[55]"=w254:sgl, "[56]"=w255:sgl)
              n240 = shared-variable "My Computer\\Instructor.lvlib\\FM-20_S"(w252) -> ()  [unwired: 1 in, 1 out]
              n241 = shared-variable "My Computer\\Instructor.lvlib\\FM-30_S"(w253) -> ()  [unwired: 1 in, 1 out]
              n242 = shared-variable "My Computer\\Instructor.lvlib\\FM-40_S"(w254) -> ()  [unwired: 1 in, 1 out]
              n243 = shared-variable "My Computer\\Instructor.lvlib\\FM-60_S"(w255) -> ()  [unwired: 1 in, 1 out]
            }
            frame "ns=2;s=Heater Res Gen" {
              n244 = Variant To Data(type=0.0, Variant=w259) -> (data=w260:dbl)  [unwired: 1 in, 1 out]
              n245 = shared-variable "My Computer\\Instructor.lvlib\\Heater Res Gen"(w260) -> ()  [unwired: 1 in, 1 out]
            }
            frame "ns=2;s=CTAH Res Gen" {
              n246 = Variant To Data(type=0.0, Variant=w262) -> (data=w263:dbl)  [unwired: 1 in, 1 out]
              n247 = shared-variable "My Computer\\Instructor.lvlib\\CTAH Res Gen"(w263) -> ()  [unwired: 1 in, 1 out]
            }
            frame "ns=2;s=CTAH Temp In Res Gen" {
              n248 = Variant To Data(type=0.0, Variant=w265) -> (data=w266:dbl)  [unwired: 1 in, 1 out]
              n249 = shared-variable "My Computer\\Instructor.lvlib\\CTAH Temp In Res Gen"(w266) -> ()  [unwired: 1 in, 1 out]
            }
            frame "ns=2;s=DHX Temp Out Res Gen" {
              n250 = Variant To Data(type=0.0, Variant=w268) -> (data=w269:dbl)  [unwired: 1 in, 1 out]
              n251 = shared-variable "My Computer\\Instructor.lvlib\\DHX Temp Out Res Gen"(w269) -> ()  [unwired: 1 in, 1 out]
            }
            frame "ns=2;s=Heater Temp Out Res Gen" {
              n252 = Variant To Data(type=0.0, Variant=w271) -> (data=w272:dbl)  [unwired: 1 in, 1 out]
              n253 = shared-variable "My Computer\\Instructor.lvlib\\Heater Temp Out Res Gen"(w272) -> ()  [unwired: 1 in, 1 out]
            }
            frame "ns=2;s=TCHX Temp In Res Gen" {
              n254 = Variant To Data(type=0.0, Variant=w274) -> (data=w275:dbl)  [unwired: 1 in, 1 out]
              n255 = shared-variable "My Computer\\Instructor.lvlib\\TCHX Temp In Res Gen"(w275) -> ()  [unwired: 1 in, 1 out]
            }
          }
        }
      }
    }
    n256 = Wait (ms)(milliseconds to wait=u32 100) -> ()  [unwired: 1 out]
    n257 = Unbundle By Name(w24) -> ("status"=w29:bool)
    n258 = Not(x=w29) -> (.not. x?=w30:bool)
    n259 = shared-variable "My Computer\\Instructor.lvlib\\Read Connection"(w30) -> ()  [unwired: 1 in, 1 out]
    n260 = shared-variable "My Computer\\Instructor.lvlib\\Stop Reading"() -> (w27:bool)  [unwired: 1 in, 1 out]
    n261 = Build Array(w29, "stop", w27) -> (w26:bool[])
    n262 = Or Array Elements(Boolean array=w26) -> (logical OR=w25:bool)
  }
  n263 = shared-variable "My Computer\\Instructor.lvlib\\Stop Reading"(w4) -> ()  [unwired: 1 in, 1 out]
  n264 = call <vilib>:"Delete Monitored Nodes.vi"("error in (no error)"=w1, "node IDs"=w7, "subscription ID in"=w11, "OPC UA client refnum in"=w6) -> ("error out"=w12:errorcluster, "OPC UA client refnum out"=w13:T4)  [unwired: 3 in, 3 out]
  n265 = Build Array(w11) -> (w10:T5[])
  n266 = call <vilib>:"Delete Subscriptions.vi"("error in (no error)"=w12, "subscription IDs"=w10, "OPC UA client refnum in"=w13) -> ("error out"=w14:errorcluster, "OPC UA client refnum out"=w15:T4)  [unwired: 6 in, 1 out]
  n267 = call <vilib>:"Disconnect.vi"("error in (no error)"=w14, "OPC UA client refnum in"=w15) -> ("error out"=→"error out":errorcluster)  [unwired: 9 in]
